vi "污染物CP编码.vi"(6 "字符串":string="N", 7 "字段结束":bool=TRUE, 8 "数据类型":string(combo)="-Rtd=", 9 "污染物浓度":string, 10 "污染物编码":string) -> (3 "编码输出":string)   [LabVIEW 2016]
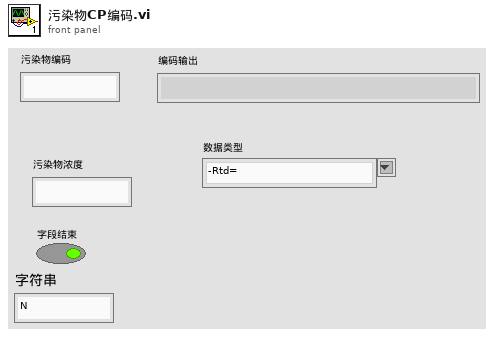
[diagram p1: front panel]
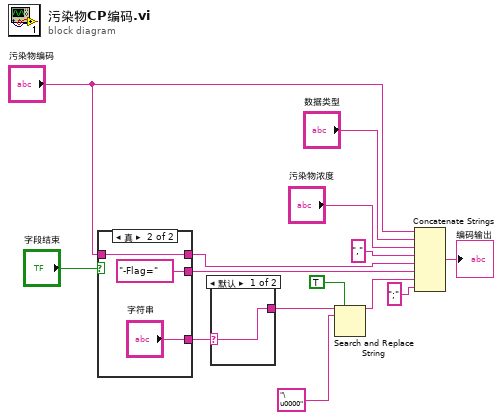
[diagram p0: block diagram]
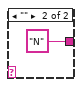
[diagram p2: hidden frame]
diagram:
  n1 = case shown="真" "字段结束" {
    tunnel: [_ "-Flag=" ("字符串")] -> w10
    tunnel: [_ "字符串"] -> w5
    tunnel: "污染物编码" -> [_ w16]
    tunnel: [_ w16] -> w7
    frame False {
    }
    frame True {
    }
  }
  n2 = case shown="默认" w5 {
    selector: w5 -> [w18 _]
    tunnel: [w18 "N" ("字符串")] -> w4
    frame Default {
    }
    frame "" {
    }
  }
  n3 = Search and Replace String(replace all?=TRUE ("替换全部？(F)"), input string=w4, search string="\u0000" ("搜索字符串")) -> (result string=w2:string)  [unwired: 5 in, 3 out]
  n4 = Concatenate Strings("污染物编码", "数据类型", "污染物浓度", "," ("字符串"), w7, w10, w2, ";" ("字符串")) -> (→"编码输出":string)
